vi "MWC INIT.vi"   [LabVIEW 2009]
uses:
  MWC Global.vi
  <vilib>/Utility/config.llb/Read Key (String).vi
  <vilib>/Utility/config.llb/Read Key (I32).vi
  TPS Global.vi
  <vilib>/Utility/config.llb/NI_LVConfig.lvlib
types:
  T1 = typedef "NI_LVConfig.lvlib/Config Data RefNum.ctl" = refnum<k1>
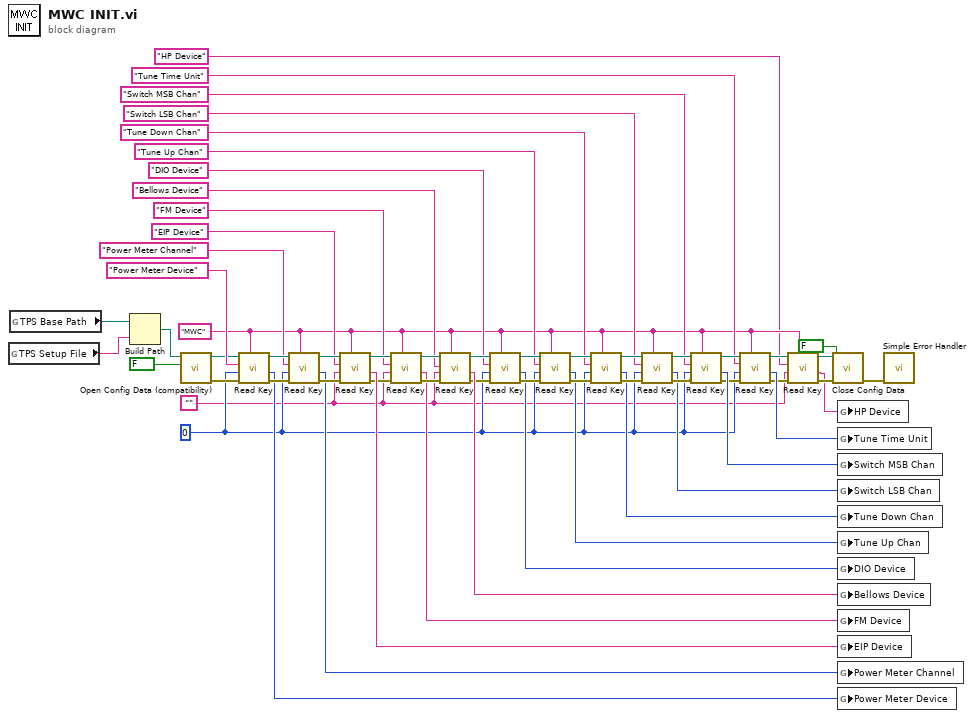
[diagram p0: block diagram]
diagram:
  w12 = 0
  w4 = ""
  w3 = "MWC" ("section")
  n1 = global read "TPS Global.vi" "TPS Setup File"() -> (w57:string)
  n2 = global read "TPS Global.vi" "TPS Base Path"() -> (w52:path)
  n3 = Build Path(base path=w52, name or relative path=w57) -> (appended path=w56:path)
  n4 = call <vilib>:"Open Config Data (compatibility).vi"("create file if necessary (T)"=FALSE ("create file if necessary? (T)"), "configuration file path"=w56) -> ("error out"=w54:errorcluster, "refnum"=w53:T1)  [unwired: 7 in, 1 out]
  n5 = call-poly <vilib>:"Read Key.vi"("section"=w3, "error in (no error)"=w54, "default value"=w12, "key"="Power Meter Device", "refnum"=w53) -> ("error out"=w51:errorcluster, "value"=w43:i32, "refnum out"=w50:T1)  [unwired: 3 in, 1 out]
  n6 = call-poly <vilib>:"Read Key.vi"("section"=w3, "error in (no error)"=w51, "default value"=w12, "key"="Power Meter Channel", "refnum"=w50) -> ("error out"=w49:errorcluster, "value"=w44:i32, "refnum out"=w48:T1)  [unwired: 3 in, 1 out]
  n7 = call-poly <vilib>:"Read Key.vi"("section"=w3, "error in (no error)"=w49, "default value"=w4, "key"="EIP Device", "refnum"=w48) -> ("error out"=w42:errorcluster, "value"=w45:string, "refnum out"=w41:T1)  [unwired: 3 in, 1 out]
  n8 = call-poly <vilib>:"Read Key.vi"("section"=w3, "error in (no error)"=w42, "default value"=w4, "key"="FM Device", "refnum"=w41) -> ("error out"=w39:errorcluster, "value"=w36:string, "refnum out"=w38:T1)  [unwired: 3 in, 1 out]
  n9 = call-poly <vilib>:"Read Key.vi"("section"=w3, "error in (no error)"=w39, "default value"=w4, "key"="Bellows Device", "refnum"=w38) -> ("error out"=w34:errorcluster, "value"=w35:string, "refnum out"=w33:T1)  [unwired: 3 in, 1 out]
  n10 = call-poly <vilib>:"Read Key.vi"("section"=w3, "error in (no error)"=w34, "default value"=w12, "key"="DIO Device", "refnum"=w33) -> ("error out"=w32:errorcluster, "value"=w24:i32, "refnum out"=w25:T1)  [unwired: 3 in, 1 out]
  n11 = call-poly <vilib>:"Read Key.vi"("section"=w3, "error in (no error)"=w32, "default value"=w12, "key"="Tune Up Chan", "refnum"=w25) -> ("error out"=w31:errorcluster, "value"=w23:i32, "refnum out"=w26:T1)  [unwired: 3 in, 1 out]
  n12 = call-poly <vilib>:"Read Key.vi"("section"=w3, "error in (no error)"=w31, "default value"=w12, "key"="Tune Down Chan", "refnum"=w26) -> ("error out"=w30:errorcluster, "value"=w22:i32, "refnum out"=w27:T1)  [unwired: 3 in, 1 out]
  n13 = call-poly <vilib>:"Read Key.vi"("section"=w3, "error in (no error)"=w30, "default value"=w12, "key"="Switch LSB Chan", "refnum"=w27) -> ("error out"=w29:errorcluster, "value"=w21:i32, "refnum out"=w28:T1)  [unwired: 3 in, 1 out]
  n14 = call-poly <vilib>:"Read Key.vi"("section"=w3, "error in (no error)"=w29, "default value"=w12, "key"="Switch MSB Chan", "refnum"=w28) -> ("error out"=w14:errorcluster, "value"=w20:i32, "refnum out"=w13:T1)  [unwired: 3 in, 1 out]
  n15 = call-poly <vilib>:"Read Key.vi"("section"=w3, "error in (no error)"=w14, "default value"=w12, "key"="Tune Time Unit", "refnum"=w13) -> ("error out"=w9:errorcluster, "value"=w10:i32, "refnum out"=w8:T1)  [unwired: 3 in, 1 out]
  n16 = call-poly <vilib>:"Read Key.vi"("section"=w3, "error in (no error)"=w9, "default value"=w4, "key"="HP Device", "refnum"=w8) -> ("error out"=w7:errorcluster, "value"=w5:string, "refnum out"=w6:T1)  [unwired: 3 in, 1 out]
  n17 = call <vilib>:"Close Config Data.vi"("error in (no error)"=w7, "write file if changed (T)"=FALSE, "refnum"=w6) -> ("error out"=w59:errorcluster)  [unwired: 7 in, 1 out]
  n18 = global write "MWC Global.vi" "HP Device"(w5) -> ()
  n19 = global write "MWC Global.vi" "Tune Time Unit"(w10) -> ()
  n20 = global write "MWC Global.vi" "Switch MSB Chan"(w20) -> ()
  n21 = global write "MWC Global.vi" "Switch LSB Chan"(w21) -> ()
  n22 = global write "MWC Global.vi" "Tune Down Chan"(w22) -> ()
  n23 = global write "MWC Global.vi" "Tune Up Chan"(w23) -> ()
  n24 = global write "MWC Global.vi" "DIO Device"(w24) -> ()
  n25 = global write "MWC Global.vi" "Bellows Device"(w35) -> ()
  n26 = global write "MWC Global.vi" "FM Device"(w36) -> ()
  n27 = global write "MWC Global.vi" "EIP Device"(w45) -> ()
  n28 = global write "MWC Global.vi" "Power Meter Channel"(w44) -> ()
  n29 = global write "MWC Global.vi" "Power Meter Device"(w43) -> ()
  n30 = call <vilib>:"Simple Error Handler.vi"("error in (no error)"=w59) -> ()  [unwired: 4 in, 5 out]
